vi "DHTxx .so Path.vi"() -> (1 "DHTxx .so Path":path=path "libdht.so")   [LabVIEW 2014, in "QwaveSys Raspberry Pi Library.lvlib"]
uses:
  QwaveSys Raspberry Pi Library.lvlib
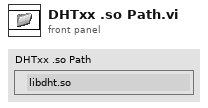
[diagram p1: front panel]
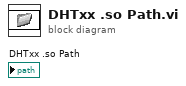
[diagram p0: block diagram]
diagram:
